vi "Vector Norm.vi"   [LabVIEW 2014, in "NI_AALPro.lvlib"]
doc: "Computes the <B>norm</B> of <B>Input Vector</B>. Wire data to the <B>Input Vector</B> input to determine the polymorphic instance to use or manually select the instance."
uses:
  NI_AALPro.lvlib
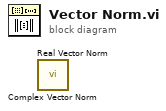
[diagram p0: block diagram]
diagram:
  n1 = call "Complex Vector Norm.vi"() -> ()  [unwired: 10 in, 2 out]
  n2 = call "Real Vector Norm.vi"() -> ()  [unwired: 10 in, 2 out]
